vi "addCheckOUT.vi"(0 "reference in":refnum<class "Project Panels.lvclass">=refnum, 11 "error in (no error)":errorcluster) -> (4 "reference out":refnum<class "Project Panels.lvclass">, 8 "saved?":bool, 15 "error out":errorcluster={"status"=TRUE, "code"=1556, "source"="In Place Element Structure in Project Panels.lvclass:addCheckIN.vi"})   [LabVIEW 2015, in "Project Panels.lvclass"]
uses:
  Project Panels.lvclass
  <vilib>/Utility/miscctls.llb/LVRowAndColumnTypeDef.ctl
  deviceState.ctl
  SYS/Items Controller_llb/Items Controller.lvclass
panel:
  out "Cell Position":T1={"Row"=0, "Column"=4}
  out "title":string="Add Check OUT"
  in  "updateData":bool
  in  "Quantity":i32
  in  "Description:":string
  in  "S/N:":string caption="Add more than one seprated by a \",\" without space"
  in  "P/N:":string
  out "dataIN":string[][](table)
  in  "Date OUT:":string caption="(dd/mm/yyyy)"
  in  "Note:":string
  in  "ADD":bool
  out "Status bar":string="Fill in all and press the DONE button....."
  in  "Stop Button":bool
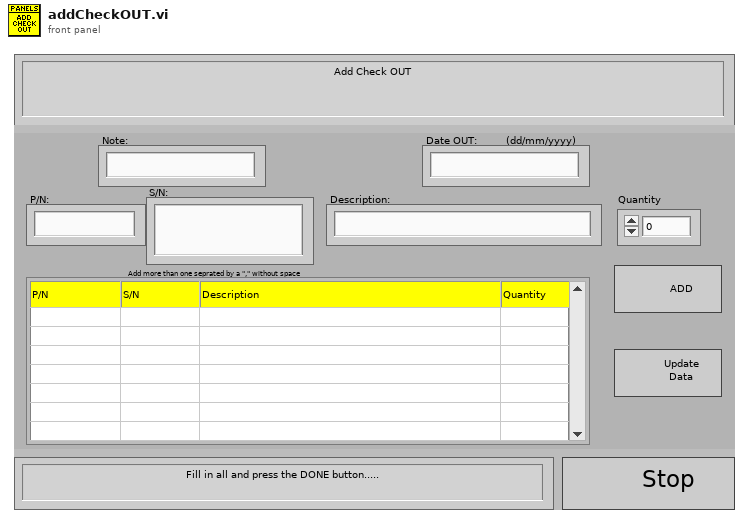
[diagram p1: front panel]
types:
  T1 = typedef "LVRowAndColumnTypeDef.ctl" = cluster{"Row":i32, "Column":i32}
  T2 = cluster{"P/N":string, "S/N":string, "Description":string, "Quantity":i32}
  T3 = typedef "Project Panels.lvclass/deviceState.ctl" = enum16{"check", "initiate", "waitEvent", "dataFromPDF", "getDetails", "save", "close", "stop"}
  T4 = typedef "Project Panels.lvclass/ObjectAttributesRef.ctl" = refnum<data-value>
  T5 = typedef "Project Panels.lvclass/ObjectAttributes.ctl" = cluster{"MyAttribute":dbl, "device_controller_ref":refnum<class "Devices Controller.lvclass">, "file_controller_ref":refnum<class "File Controller.lvclass">, "item_controller_ref":refnum<class "Items Controller.lvclass">, "item_tables":cluster{"checkIN":string[][], "checkOUT":string[][], "storage":string[][]}, "quickbook_table":cluster{"notes":string[][]}, "notification_controller_ref":refnum<class "Notification Controller.lvclass">, "partstracking_controller_ref":refnum<class "PartsTracking Controller.lvclass">, "product_tables":cluster{"k4b2":string[][], "fitmate":string[][], "RMR":string[][], "CPET":string[][], "BP":string[][], "PP":string[][], "k5":string[][], "bb-pft":string[][]}, "rowsColour":u32[]}
  T6 = typedef "LVPoint32TypeDef.ctl" = cluster{"Horizontal":i32, "Vertical":i32}
  T7 = enum16{"Left Button", "Center Button", "Right Button", "Window Close"}
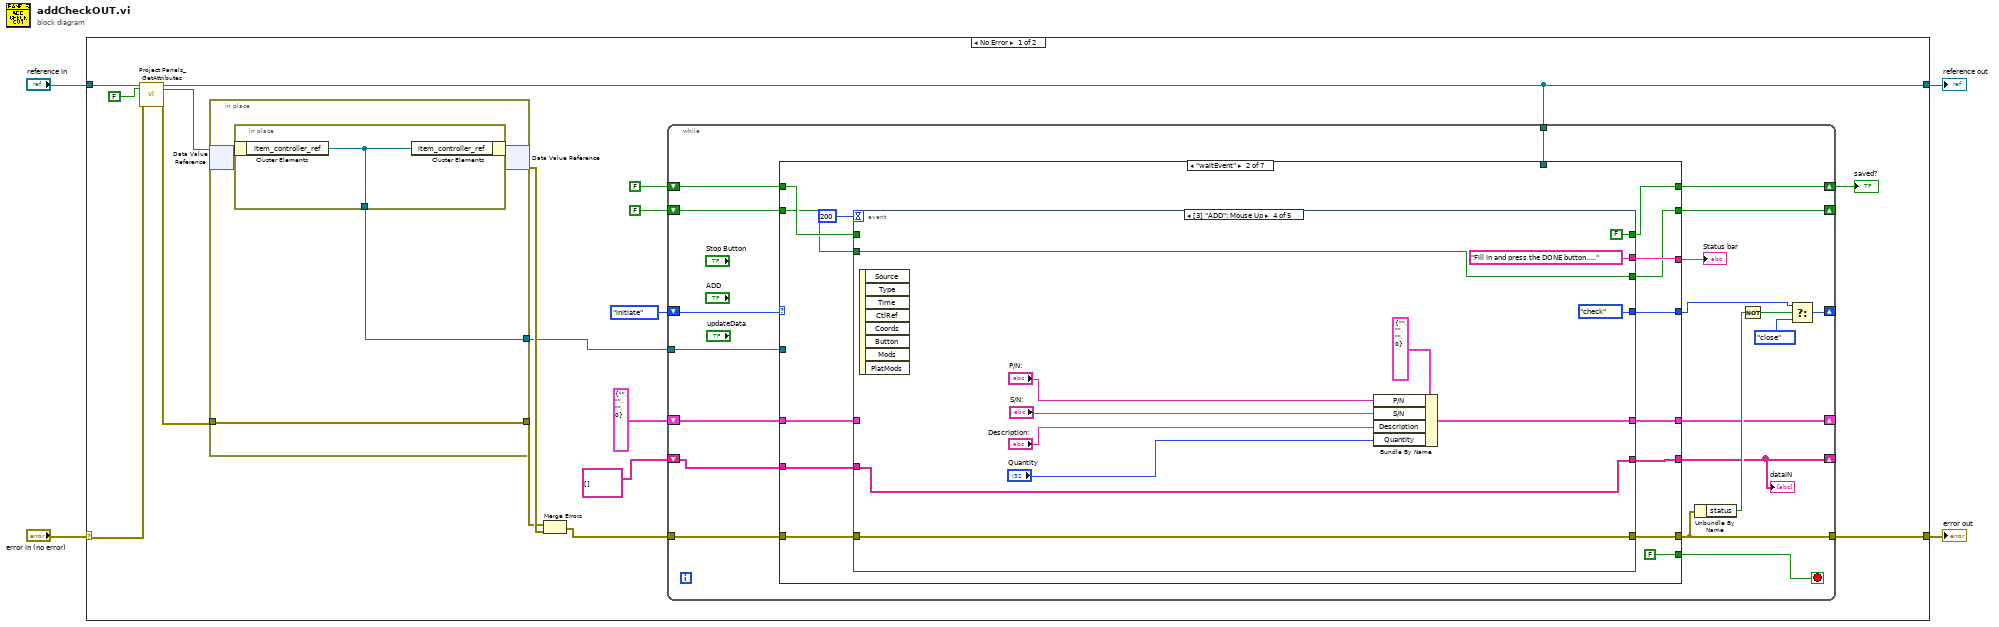
[diagram p0: block diagram]
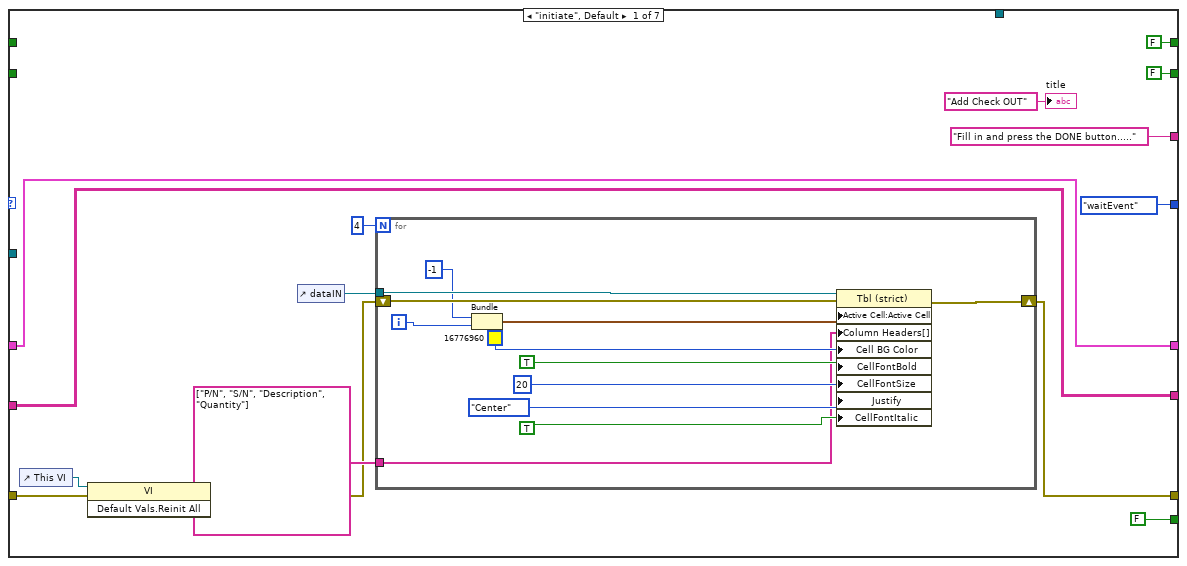
[diagram p2: hidden frame]
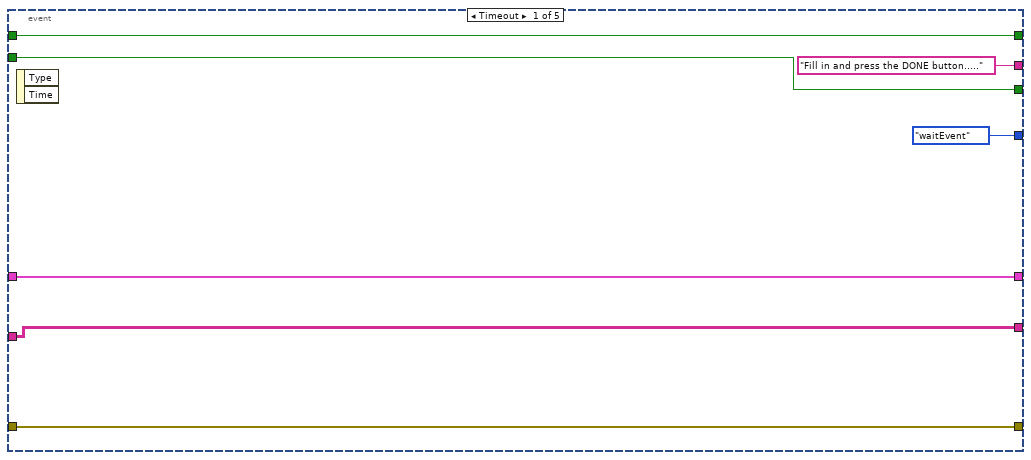
[diagram p3: hidden frame]
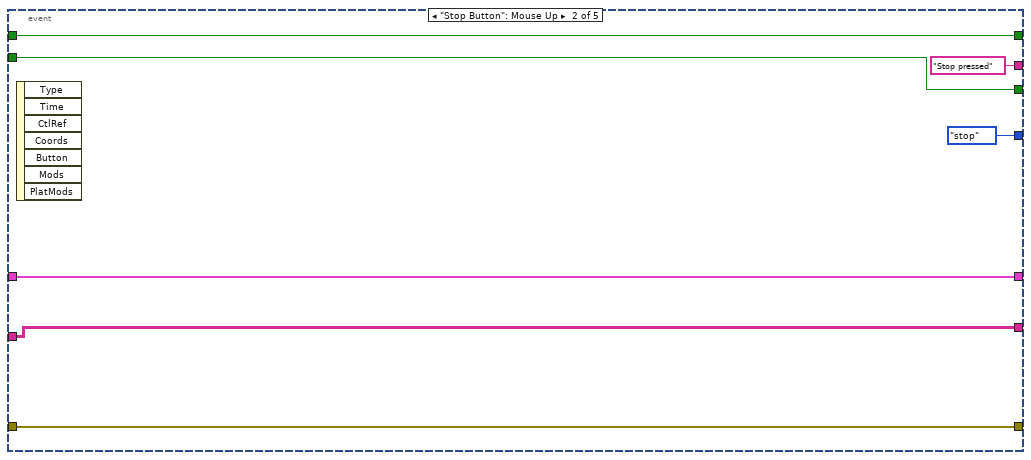
[diagram p4: hidden frame]
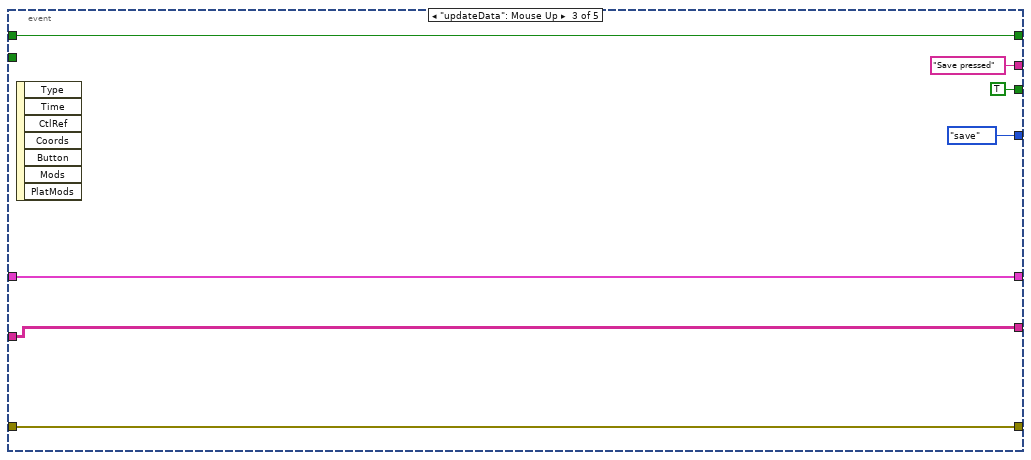
[diagram p5: hidden frame]
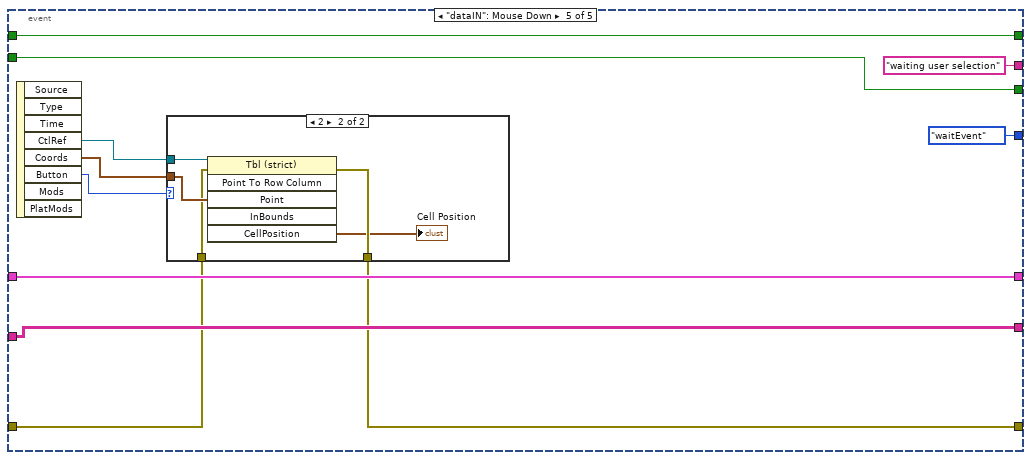
[diagram p6: hidden frame]
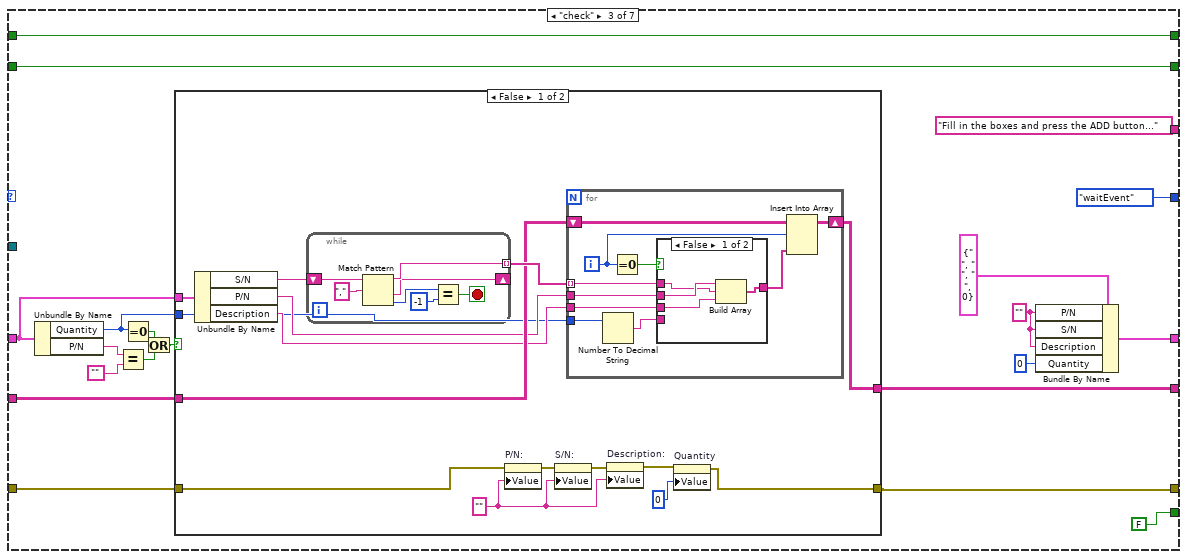
[diagram p8: hidden frame]
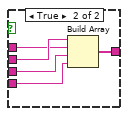
[diagram p9: hidden frame]
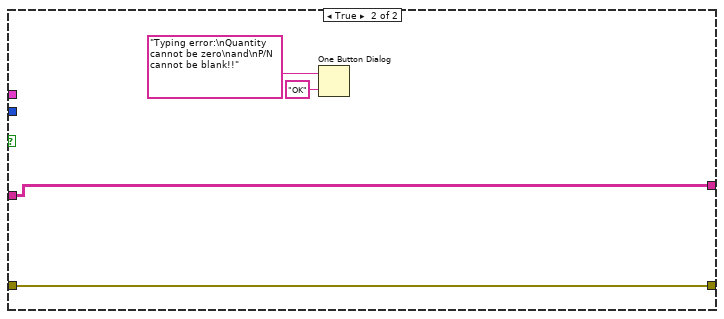
[diagram p10: hidden frame]
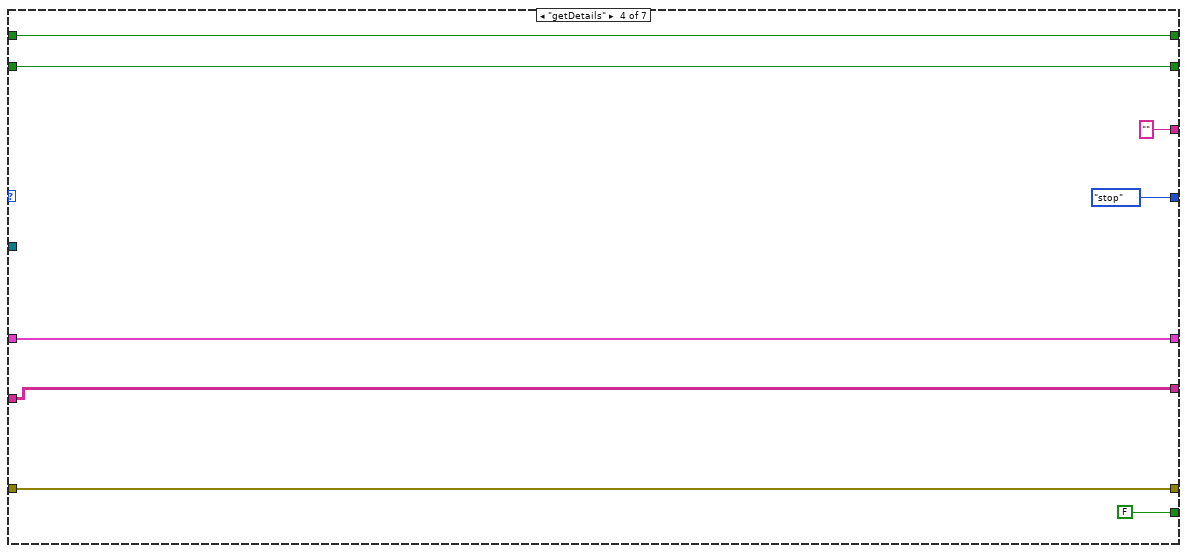
[diagram p11: hidden frame]
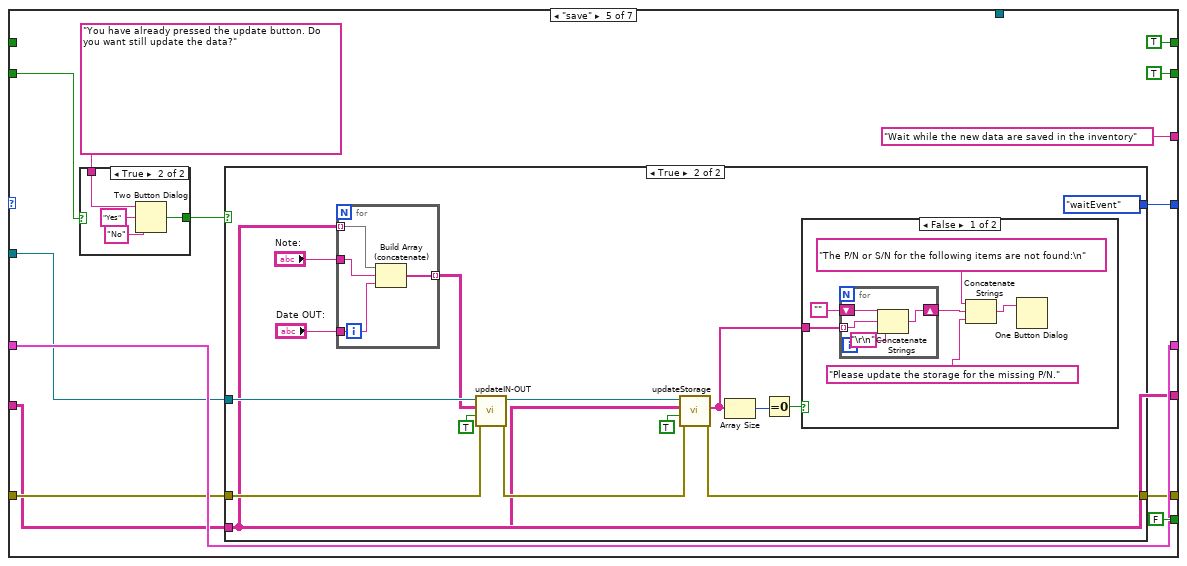
[diagram p12: hidden frame]
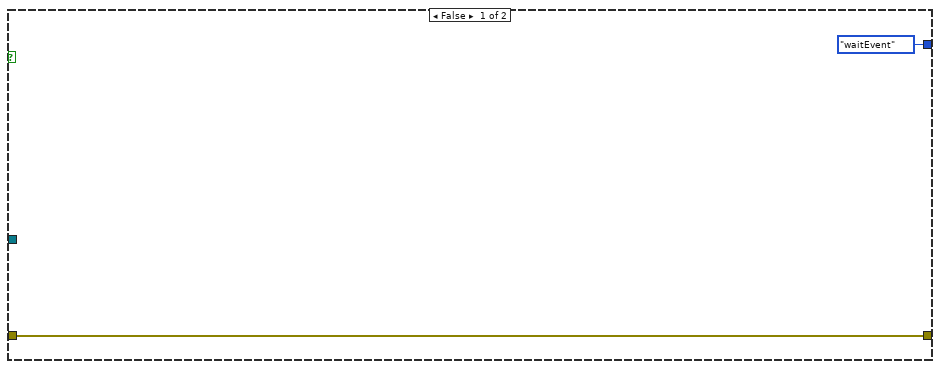
[diagram p13: hidden frame]
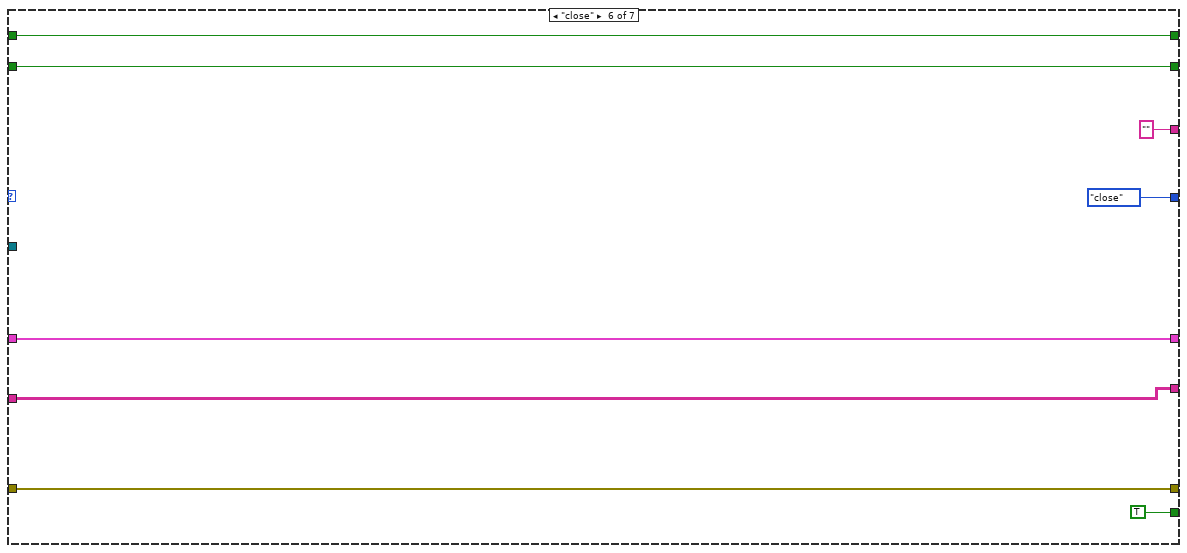
[diagram p16: hidden frame]
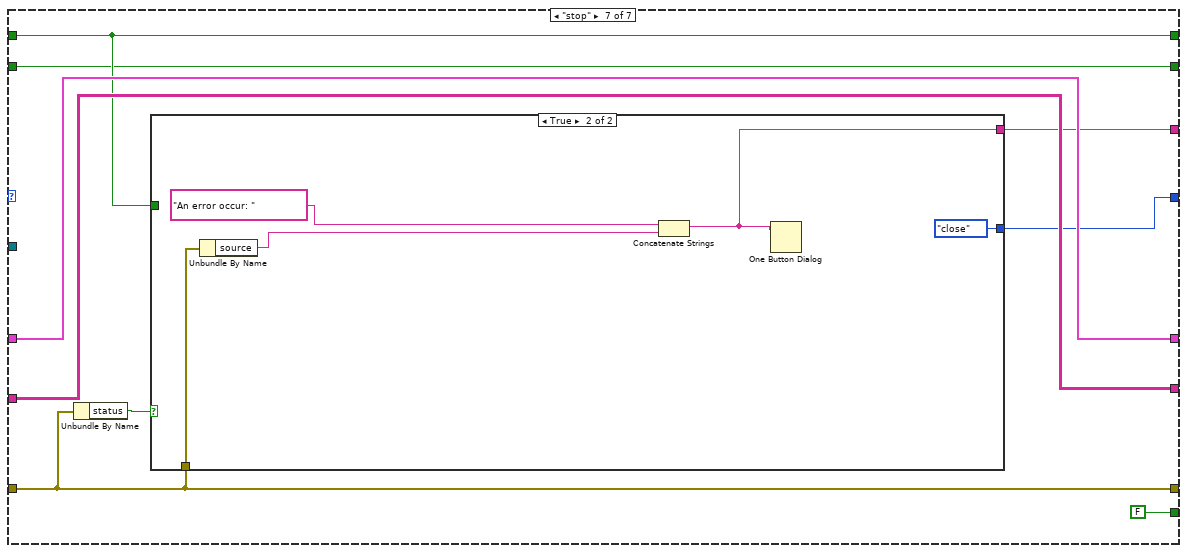
[diagram p17: hidden frame]
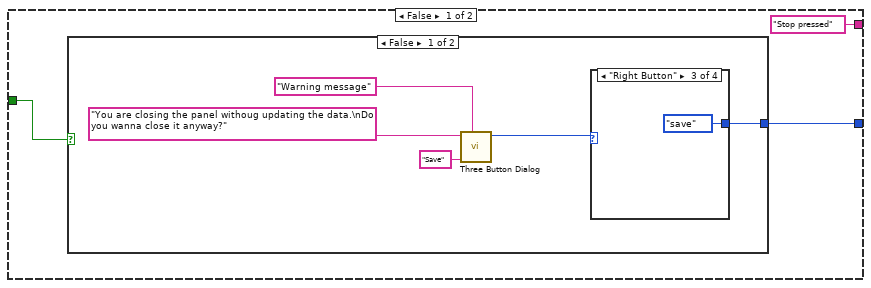
[diagram p18: hidden frame]
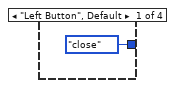
[diagram p19: hidden frame]
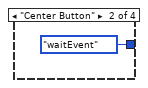
[diagram p20: hidden frame]
diagram:
  n1 = case shown="No Error" "error in (no error)" {
    selector: "error in (no error)" -> [w17 w296]
    tunnel: [w14 w296] -> w3
    tunnel: [w12 w295] -> w1
    tunnel: "reference in" -> [w19 w295]
    frame No Error {
      n2 = call "Project Panels_GetAttributes.vi"("reference in"=w19, "return data? (T)"=FALSE, "error in (no error)"=w17) -> ("reference out"=w12:refnum<class "Project Panels.lvclass">, "attributes ref"=w15:T4, "error out"=w16:errorcluster)  [unwired: 13 in, 1 out]
      n3 = in-place {
        in-place-border: w16 -> [w291]
        in-place-border: [w291] -> w20
        in-place-border: [w290] -> w10
        n4 = in-place-dvr #1(w15) -> (w292:T5)  [unwired: 1 out]
        n5 = in-place {
          in-place-border: [w294] -> w290
          n6 = in-place-cluster #2(w292) -> ("item_controller_ref"=w294:refnum<class "Items Controller.lvclass">)
          n7 = in-place-cluster #2("item_controller_ref"=w294) -> (w293:T5)
        }
        n8 = in-place-dvr #1(w293) -> (w21:errorcluster)  [unwired: 1 out]
      }
      n9 = Merge Errors(w20, w21) -> (w11:errorcluster)
      n10 = while {
        tunnel: w11 -> [w41]
        tunnel: [w37] -> w14
        shift-right: [w38] -> _
        shift-left: deviceState."initiate" ("state") -> [w40]
        tunnel: w12 -> [w33]
        tunnel: w10 -> [w31]
        shift-right: [w29] -> _
        shift-left: T2 {"P/N"="", "S/N"="", "Description"="", "Quantity"=0} -> [w28]
        shift-right: [w27] -> _
        shift-left: string[][] [] ("dataIN 2") -> [w26]
        shift-right: [w24] -> w6
        shift-left: FALSE -> [w25]
        shift-right: [w22] -> _
        shift-left: FALSE -> [w23]
        stop <- w32 stop-if-true
        n11 = case shown="\"waitEvent\"" w40 {
          tunnel: w41 -> [w52 w82 w149 w204 w213 w261 w269]
          tunnel: [w47 w81 w140 w204 w212 w261 w269] -> w37
          tunnel: [deviceState."waitEvent" ("state") w79 deviceState."waitEvent" ("f") deviceState."stop" ("f") w218 deviceState."close" ("f") w265] -> w39
          tunnel: w33 -> [_ _ _ _ _ _ _]
          tunnel: [FALSE FALSE FALSE FALSE FALSE TRUE FALSE] -> w32
          tunnel: w31 -> [_ _ _ _ w214 _ _]
          tunnel: ["Fill in and press the DONE button....." ("Status bar") w77 "Fill in the boxes and press the ADD button..." ("Status bar") "" ("Status bar") "Wait while the new data are saved in the inventory" ("Status bar") "" ("Status bar") w266] -> w30
          tunnel: [w45 w76 w143 w201 w215 w258 w268] -> w29
          tunnel: w28 -> [w45 w75 w145 w201 w215 w258 w268]
          tunnel: w26 -> [w44 w74 w148 w200 w210 w257 w267]
          tunnel: [w44 w73 w147 w200 w210 w257 w267] -> w27
          tunnel: w25 -> [_ w72 w139 w199 _ w256 w264]
          tunnel: [FALSE w71 w139 w199 TRUE w256 w264] -> w24
          tunnel: w23 -> [_ w70 w133 w198 w209 w255 w263]
          tunnel: [FALSE w69 w133 w198 TRUE w255 w263] -> w22
          frame "initiate", Default {
            n12 = control-ref of="This VI"() -> (w53:refnum<vi>)
            n13 = invoke class="VI" method="Default Vals.Reinit All"(reference=w53, error in=w52) -> (error out=w48:errorcluster)  [unwired: 1 in, 2 out]
            n14 = control-ref of="dataIN"() -> (w49:refnum<vi>)
            n15 = for {
              N: 4 -> [_]
              tunnel: w49 -> [w66]
              shift-right: [w67] -> w47
              shift-left: w48 -> [w68]
              tunnel: string[] ["P/N", "S/N", "Description", "Quantity"] ("Column Header Strings[]") -> [w57]
              i -> [w64]
              n16 = Bundle("index"=-1, w64) -> (w65:cluster{"index":i32, i32})  [unwired: 1 in]
              n17 = property on="Property Node" class="Tbl (strict)"(reference=w66, error in=w68, "Active Cell:Active Cell"=w65, "Column Headers[]"=w57, "Cell BG Color"=u32 16776960, "CellFontBold"=TRUE ("Active Cell:Cell Font:Bold"), "CellFontSize"=u32 20 ("Active Cell:Cell Font:Size"), "Justify"=enum16{"Left", "Center", "Right"}."Center" ("Active Cell:Cell Justification"), "CellFontItalic"=TRUE ("Active Cell:Cell Font:Italic")) -> (error out=w67:errorcluster)  [unwired: 1 out]
            }
            "title" <- "Add Check OUT" ("title")
          }
          frame "waitEvent" {
            n18 = event shown="[3] \"ADD\": Mouse Up" {
              selector: _ -> [_ _ _ _ _]
              dyn-events: _ -> [_ _ _ _ _]
              timeout: 200 -> [_ _ _ _ _]
              tunnel: w82 -> [w89 w95 w102 w115 w118]
              tunnel: [w89 w95 w102 w115 w117] -> w81
              tunnel: [deviceState."waitEvent" ("f") deviceState."stop" ("f") deviceState."save" ("f") deviceState."check" ("f") deviceState."waitEvent" ("f")] -> w79
              tunnel: ["Fill in and press the DONE button....." ("Status bar") "Stop pressed" ("Status bar") "Save pressed" ("Status bar") "Fill in and press the DONE button....." ("Status bar") "waiting user selection" ("Status bar")] -> w77
              tunnel: [w86 w93 w100 w109 w122] -> w76
              tunnel: w75 -> [w86 w93 w100 _ w122]
              tunnel: w74 -> [w85 w92 w99 w106 w123]
              tunnel: [w85 w92 w99 w106 w123] -> w73
              tunnel: w72 -> [w84 w91 w98 _ w126]
              tunnel: [w84 w91 w98 FALSE w126] -> w71
              tunnel: w70 -> [w83 w90 _ w104 w124]
              tunnel: [w83 w90 TRUE w104 w124] -> w69
              event Timeout {
                n19 = event-data() -> ()  [unwired: 1 in, 2 out]
              }
              event "Stop Button": Mouse Up {
                n20 = event-data() -> ()  [unwired: 1 in, 7 out]
              }
              event "updateData": Mouse Up {
                n21 = event-data() -> ()  [unwired: 1 in, 7 out]
              }
              event "ADD": Mouse Up {
                n22 = event-data() -> ()  [unwired: 1 in, 8 out]
                n23 = Bundle By Name(cluster=T2 {"P/N"="", "S/N"="", "Description"="", "Quantity"=0}, "P/N"="P/N:", "S/N"="S/N:", "Description"="Description:", "Quantity"="Quantity") -> (w109:T2)
              }
              event "dataIN": Mouse Down {
                n24 = event-data() -> ("CtlRef"=w119:refnum<vi>, "Coords"=w120:T6, "Button"=w121:u16)  [unwired: 1 in, 5 out]
                n25 = case shown="2" w121 {
                  tunnel: w119 -> [_ w132]
                  tunnel: w120 -> [_ w131]
                  tunnel: w118 -> [w127 w130]
                  tunnel: [w127 w129] -> w117
                  frame 0, Default {
                  }
                  frame 2 {
                    n26 = invoke class="Tbl (strict)" method="Point To Row Column"(reference=w132, error in=w130, "Point"=w131) -> (error out=w129:errorcluster, "CellPosition"=→"Cell Position":T1)  [unwired: 3 in, 4 out]
                  }
                }
              }
            }
          }
          frame "check" {
            w142 = "" ("P/N")
            n27 = Unbundle By Name(w145) -> ("Quantity"=w146:i32, "P/N"=w138:string)
            n28 = Equal?(x=w138, y="") -> (x = y?=w135:bool)
            n29 = Equal To 0?(x=w146) -> (x = 0?=w134:bool)
            n30 = Or(x=w134, y=w135) -> (x .or. y?=w136:bool)
            n31 = case shown="False" w136 {
              tunnel: w149 -> [w154 w197]
              tunnel: [w153 w197] -> w140
              tunnel: w148 -> [w165 w194]
              tunnel: [w160 w194] -> w147
              tunnel: w146 -> [w161 _]
              tunnel: w145 -> [w167 _]
              frame False {
                w158 = "" ("P/N:")
                n32 = Unbundle By Name(w167) -> ("S/N"=w164:string, "P/N"=w163:string, "Description"=w162:string)
                n33 = while {
                  tunnel: [w192] -> w166 mode=indexing
                  shift-right: [w188] -> _
                  shift-left: w164 -> [w187]
                  stop <- w191 stop-if-true
                  n34 = Match Pattern(string=w187, regular expression=",") -> (before substring=w192:string, after substring=w188:string, offset past match=w190:i32)  [unwired: 1 in, 1 out]
                  n35 = Equal?(x=w190, y=-1) -> (x = y?=w191:bool)
                }
                n36 = property on="P/N:" class="Str"(error in=w154, "Value"=w158) -> (error out=w155:errorcluster)  [unwired: 1 in, 1 out]
                n37 = property on="S/N:" class="Str"(error in=w155, "Value"=w158) -> (error out=w156:errorcluster)  [unwired: 1 in, 1 out]
                n38 = for {
                  tunnel: w166 -> [w176] mode=indexing
                  tunnel: w163 -> [w177]
                  tunnel: w162 -> [w175]
                  shift-right: [w173] -> w160
                  shift-left: w165 -> [w174]
                  tunnel: w161 -> [w171]
                  i -> [w168]
                  n39 = Number To Decimal String(number=w171) -> (decimal integer string=w170:string)  [unwired: 1 in]
                  n40 = Equal To 0?(x=w168) -> (x = 0?=w169:bool)
                  n41 = case shown="False" w169 {
                    tunnel: w177 -> [w179 w186]
                    tunnel: w176 -> [w178 w185]
                    tunnel: w175 -> [w180 w184]
                    tunnel: [w181 w183] -> w172
                    tunnel: w170 -> [_ w182]
                    frame False {
                      n42 = Build Array(w179, w178, w180) -> (w181:string[])
                    }
                    frame True {
                      n43 = Build Array(w186, w185, w184, w182) -> (w183:string[])
                    }
                  }
                  n44 = Insert Into Array(array=w174, index (row)=w168, new element=w172) -> (w173:string[][])  [unwired: 1 in]
                }
                n45 = property on="Description:" class="Str"(error in=w156, "Value"=w158) -> (error out=w157:errorcluster)  [unwired: 1 in, 1 out]
                n46 = property on="Quantity" class="DigNum (strict)"(error in=w157, "Value"=0 ("Quantity")) -> (error out=w153:errorcluster)  [unwired: 1 in, 1 out]
              }
              frame True {
                n47 = One Button Dialog(message="Typing error:\nQuantity cannot be zero\nand\nP/N cannot be blank!!", button name ("OK")="OK") -> ()  [unwired: 1 out]
              }
            }
            n48 = Bundle By Name(cluster=T2 {"P/N"=" ", "S/N"=" ", "Description"=" ", "Quantity"=0}, "P/N"=w142, "S/N"=w142, "Description"=w142, "Quantity"=0) -> (w143:T2)
          }
          frame "getDetails" {
          }
          frame "save" {
            n49 = case shown="True" w209 {
              selector: w209 -> [w250 _]
              tunnel: [w250 w254] -> w208
              tunnel: "You have already pressed the update button. Do you want still update the data?" ("message") -> [_ w253]
              frame False {
              }
              frame True {
                n50 = Two Button Dialog(message=w253, 1:"No" ("F button name (\"Cancel\")"), 2:"Yes" ("T button name (\"OK\")")) -> (T button?=w254:bool)
              }
            }
            n51 = case shown="True" w208 {
              tunnel: [deviceState."waitEvent" ("f") deviceState."waitEvent" ("f")] -> w218
              tunnel: w214 -> [_ w232]
              tunnel: w213 -> [w220 w231]
              tunnel: [w220 w225] -> w212
              tunnel: w210 -> [_ w221]
              frame False {
              }
              frame True {
                n52 = for {
                  tunnel: w221 -> [w246] mode=indexing
                  tunnel: "Note:" -> [w249]
                  tunnel: "Date OUT:" -> [w248]
                  tunnel: [w247] -> w228 mode=indexing
                  n53 = Build Array (concatenate)(w246, w249, w248) -> (w247:string[])
                }
                n54 = call "updateIN-OUT.vi"("error in (no error)"=w231, "IN-OUT"=TRUE, "dataIN"=w228, "reference in"=w232) -> ("error out"=w226:errorcluster, "reference out"=w229:refnum<class "Items Controller.lvclass">)  [unwired: 6 in]
                n55 = call "updateStorage.vi"("error in (no error)"=w226, "IN-OUT"=TRUE, "dataIN"=w221, "reference in"=w229) -> ("error out"=w225:errorcluster, "warningMess"=w222:string[])  [unwired: 5 in, 1 out]
                n56 = Array Size(array=w222) -> (size(s)=w224:i32)
                n57 = Equal To 0?(x=w224) -> (x = 0?=w223:bool)
                n58 = case shown="False" w223 {
                  tunnel: w222 -> [w241 _]
                  frame False {
                    n59 = for {
                      tunnel: w241 -> [w243] mode=indexing
                      shift-right: [w245] -> w239
                      shift-left: "" -> [w244]
                      n60 = Concatenate Strings(w244, w243, "\r\n") -> (w245:string)
                    }
                    n61 = Concatenate Strings("The P/N or S/N for the following items are not found:\n", w239, "Please update the storage for the missing P/N.") -> (w237:string)
                    n62 = One Button Dialog(message=w237) -> ()  [unwired: 1 in, 1 out]
                  }
                  frame True {
                  }
                }
              }
            }
          }
          frame "close" {
          }
          frame "stop" {
            n63 = Unbundle By Name(w269) -> ("status"=w270:bool)
            n64 = case shown="True" w270 {
              tunnel: w269 -> [_ w287]
              tunnel: ["Stop pressed" w286] -> w266
              tunnel: [w273 deviceState."close" ("f")] -> w265
              tunnel: w264 -> [w272 _]
              frame False {
                n65 = case shown="False" w272 {
                  tunnel: [w275 deviceState."close" ("f")] -> w273
                  frame False {
                    n66 = call <vilib>:"Three Button Dialog.vi"("Window Title (\"\")"="Warning message" ("Window Title (\"\")"), "Right Button Text (\"Cancel\")"="Save" ("Right Button Text (\"Cancel\")"), "message"="You are closing the panel withoug updating the data.\nDo you wanna close it anyway?") -> ("Which Button?"=w276:T7)  [unwired: 8 in]
                    n67 = case shown="\"Right Button\"" w276 {
                      tunnel: [deviceState."close" ("f") deviceState."waitEvent" ("f") deviceState."save" ("f") deviceState."waitEvent" ("f")] -> w275
                      frame "Left Button", Default {
                      }
                      frame "Center Button" {
                      }
                      frame "Right Button" {
                      }
                      frame "Window Close" {
                      }
                    }
                  }
                  frame True {
                  }
                }
              }
              frame True {
                n68 = Unbundle By Name(w287) -> ("source"=w288:string)
                n69 = Concatenate Strings("An error occur: " ("message"), w288) -> (w286:string)
                n70 = One Button Dialog(message=w286) -> ()  [unwired: 1 in, 1 out]
              }
            }
          }
        }
        "dataIN" <- w27
        "Status bar" <- w30
        n71 = Unbundle By Name(w37) -> ("status"=w36:bool)
        n72 = Not(x=w36) -> (.not. x?=w35:bool)
        n73 = Select(t=w39, s=w35, f=deviceState."close") -> (s? t:f=w38:T3)
      }
      "saved?" <- w6
    }
    frame Error {
    }
  }
  "error out" <- w3
  "reference out" <- w1
